vi "MGI Degrees to Radians.vi"   [LabVIEW 2020]
doc: "Convert the input degrees to radians.\n\nFreeware from Moore Good Ideas, www.mooregoodideas.com. Do not remove this line."
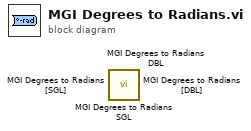
[diagram p0: block diagram]
diagram:
  n1 = call <userlib>:"MGI Degrees to Radians SGL.vi"() -> ()  [unwired: 1 in, 1 out]
  n2 = call <userlib>:"MGI Degrees to Radians DBL.vi"() -> ()  [unwired: 1 in, 1 out]
  n3 = call <userlib>:"MGI Degrees to Radians [SGL].vi"() -> ()  [unwired: 1 in, 1 out]
  n4 = call <userlib>:"MGI Degrees to Radians [DBL].vi"() -> ()  [unwired: 1 in, 1 out]
